vi "voltage.vi"(9 "u":dbl=1.0 format="%#_13g", 11 "Qube":refnum<class "Qube.lvclass">) -> (3 "Qube":refnum<class "Qube.lvclass">)   [LabVIEW 2017, in "Qube.lvclass"]
uses:
  Qube.lvclass
  <vilib>/Quanser/Rapid Control Prototyping Toolkit/hardware/HIL Board/HIL Board.lvclass
  <vilib>/Quanser/Rapid Control Prototyping Toolkit/hardware/HIL Board/_TypeSpecific/HIL Write Analog (Scalar).vi
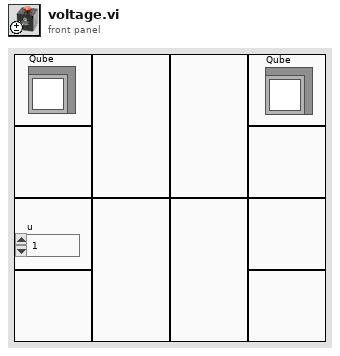
[diagram p1: front panel]
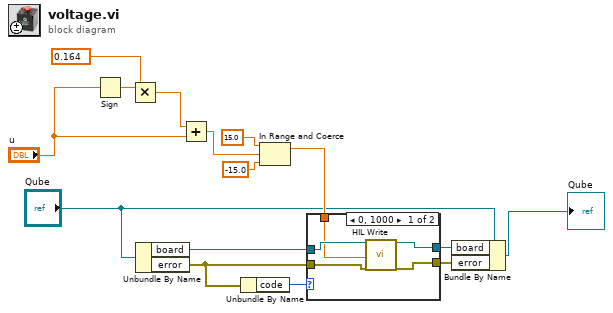
[diagram p0: block diagram]
diagram:
  n1 = Sign(1:"u") -> (0:w7:dbl)
  n2 = Multiply(x=w7, y=0.164) -> (x*y=w5:dbl)
  n3 = Unbundle By Name("Qube") -> ("board"=w15:refnum<class "HIL Board.lvclass">, "error"=w1:errorcluster)
  n4 = Add(x=w5, y="u") -> (x+y=w3:dbl)
  n5 = Unbundle By Name(w1) -> ("code"=w2:i32)
  n6 = In Range and Coerce(upper limit=15.0, x=w3, lower limit=-15.0) -> (coerced(x)=w10:dbl)  [unwired: 1 out]
  n7 = case shown="0, 1000" w2 {
    tunnel: w15 -> [w20 w22]
    tunnel: [w19 w22] -> w14
    tunnel: [w18 w21] -> w13
    tunnel: w10 -> [w17 _]
    tunnel: w1 -> [w16 w21]
    frame 0, 1000 {
      n8 = call-poly <vilib>:"HIL Write.vi"("board in"=w20, "voltage"=w17, "error in (no error)"=w16) -> ("board out"=w19:refnum<class "HIL Board.lvclass">, "error out"=w18:errorcluster)  [unwired: 15 in]
    }
    frame Default {
    }
  }
  n9 = Bundle By Name(cluster="Qube", "board"=w14, "error"=w13) -> (→"Qube":refnum<class "Qube.lvclass">)
